vi "read.vi"() -> ()   [LabVIEW 2021]
panel:
  in  "Filename":path=path "test.lvm"
  out "Waveform Graph":dynamicdata(graph)
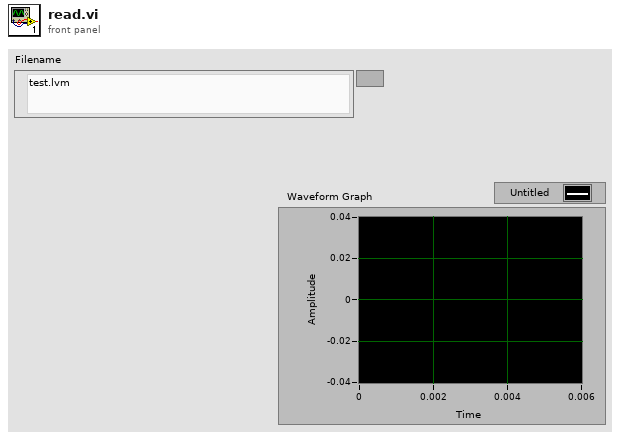
[diagram p1: front panel]
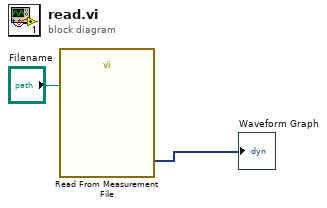
[diagram p0: block diagram]
diagram:
  n1 = call "Read From Measurement File"("Filename"="Filename") -> ("Signals"=→"Waveform Graph":dynamicdata)  [unwired: 5 in, 5 out]
